vi "MakeHotLoopCode.vi"(11 "HotTarget":dbl=40.0 min=-230.0 max=30.0) -> (3 "resulting string":string="define hotloop(while (1) {if (#3C > 40.0) {relays&=11} if (#3C < 40.0){relays|=4} pause 0.1 s })")   [LabVIEW 2023]
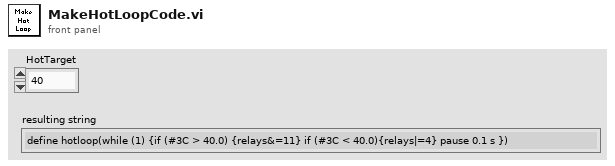
[diagram p1: front panel]
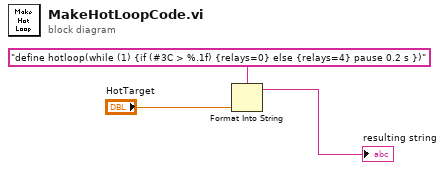
[diagram p0: block diagram]
diagram:
  n1 = Format Into String(format string="define hotloop(while (1) {if (#3C > %.1f) {relays=0} else {relays=4} pause 0.2 s })", "HotTarget") -> (resulting string=→"resulting string":string)  [unwired: 2 in, 1 out]
